vi "winchMotorCode.vi"() -> (2 "armMotorValue":dbl, 3 "elToroSplit":bool)   [LabVIEW 2013]
uses:
  <vilib>/Rock Robotics/WPI/DriverStation/WPI_DriverStationCommDataCacheOp.ctl
panel:
  in  "upperBoundDunk":dbl=16000.0
  in  "lowerBoundDunk":dbl=13000.0
  out "RawControlByte":u8 format="%08b"
  in  "upperBoundTruss":dbl=13000.0 format="%#_13g"
  in  "lowerBoundTruss":dbl=8000.0 format="%#_13g"
  in  "Encoder height shot constant":dbl=18500.0 format="%#_13g"
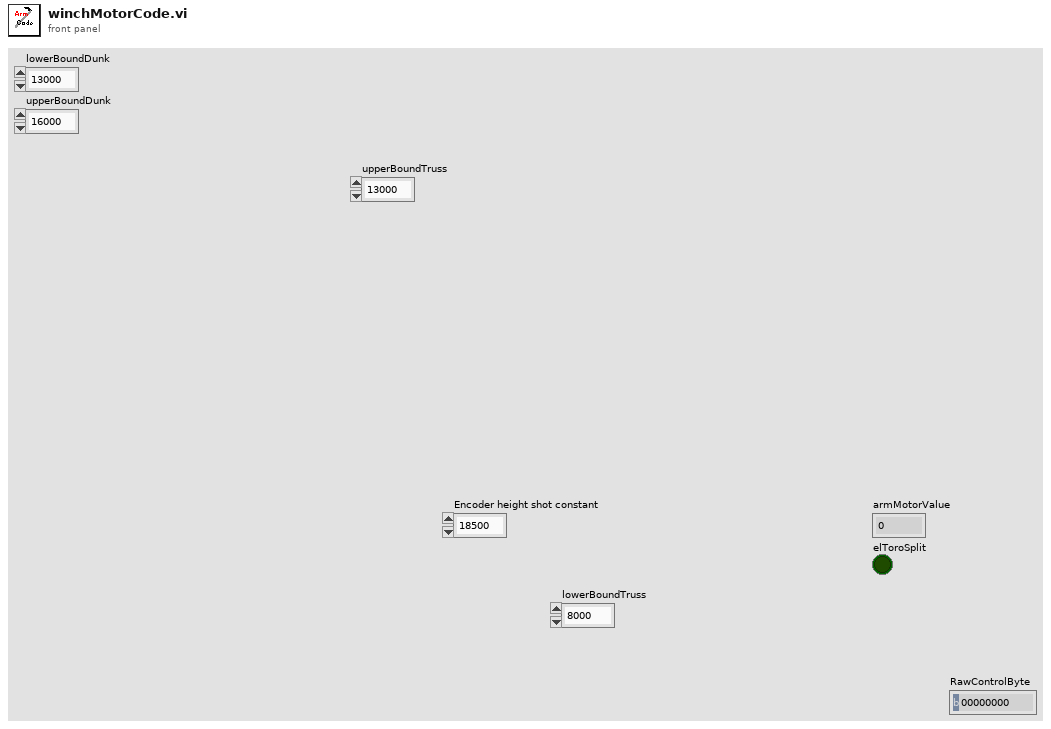
[diagram p1: front panel]
types:
  T1 = typedef "WPI_DriverStationCommDataCacheOp.ctl" = enum16{"Get", "Set", "Init"}
  T2 = typedef "WPI_EncoderDevRef.ctl" = cluster{"DevStatus":errorcluster, "EncoderIndex":T3, "CounterIndex":T4, "DistancePerCount":dbl, "Decoding Type":T5}
  T3 = typedef "FPGA_EncoderIdx.ctl" = enum8{"Enc 0", "Enc 1", "Enc 2", "Enc 3", "Invalid"}
  T4 = typedef "FPGA_CounterCtrSystemIndex.ctl" = enum8{"Ctr 0", "Ctr 1", "Ctr 2", "Ctr 3", "Ctr 4", "Ctr 5", "Ctr 6", "Ctr 7", "Invalid"}
  T5 = typedef "WPI_EncoderType.ctl" = enum16{"1x", "2x", "4x"}
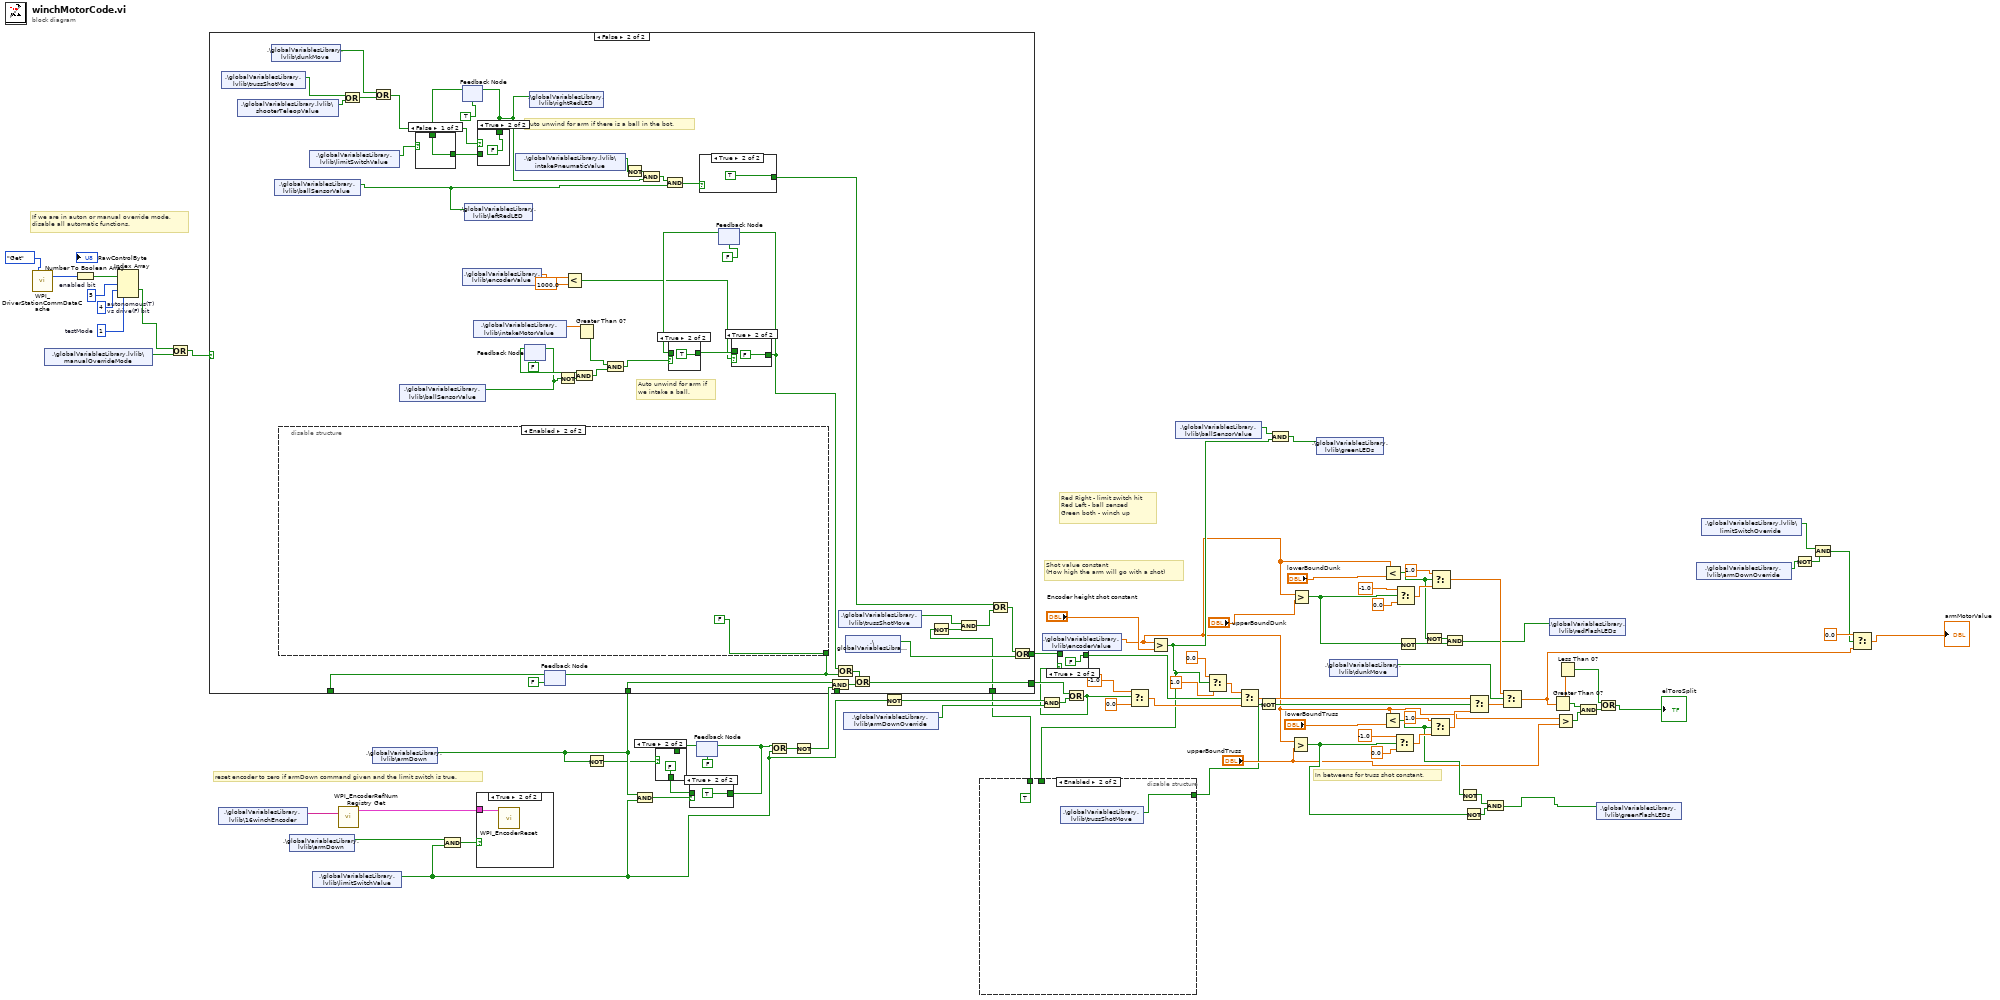
[diagram p0: block diagram]
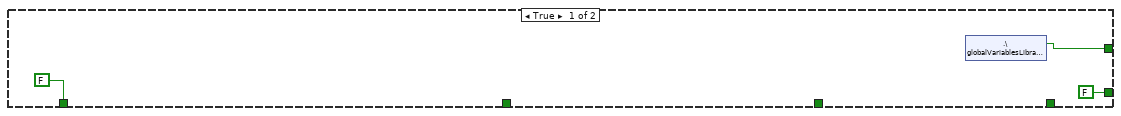
[diagram p2: hidden frame]
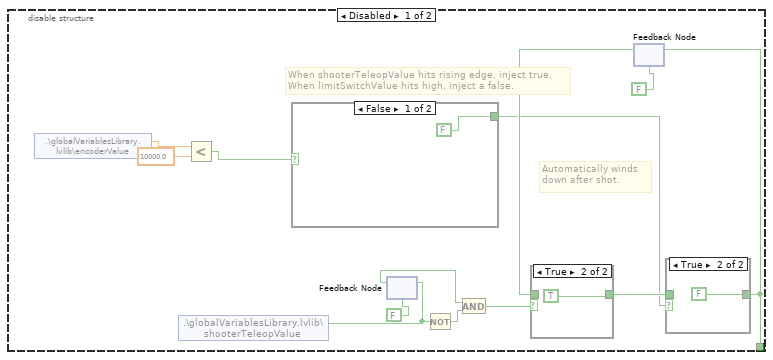
[diagram p3: hidden frame]
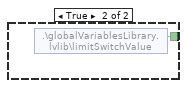
[diagram p4: hidden frame]
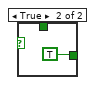
[diagram p10: hidden frame]
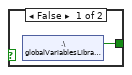
[diagram p11: hidden frame]
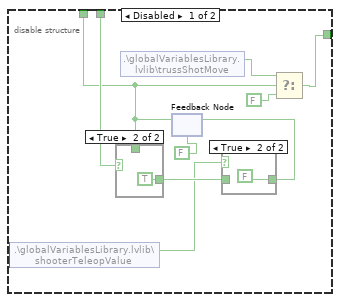
[diagram p12: hidden frame]
diagram:
  w29 = 1  # testMode
  w30 = 4  # autonomous(T) vs drive(F) bit
  w31 = 5  # enabled bit
  # "If we are in auton or manual override mode,\ndisable all automatic functions."
  # "reset encoder to zero if armDown command given and the limit switch is true."
  # "Red Right - limit switch hit\nRed Left - ball sensed\nGreen both - winch up"
  # "In betweens for truss shot constant."
  # "Shot value constant\n(How high the arm will go with a shot)"
  n1 = call <vilib>:"WPI_DriverStationCommDataCache.vi"("CommDataCacheOp"=WPI_DriverStationCommDataCacheOp."Get") -> ("ControlBit out"=w33:u8)  [unwired: 18 out]
  n2 = shared-variable ".\\globalVariablesLibrary.lvlib\\manualOverrideMode"() -> (w26:bool)  [unwired: 1 in, 1 out]
  n3 = Number To Boolean Array(number=w33) -> (Boolean array=w32:bool[])
  n4 = Index Array(array=w32, index #1=w31, index #2=w30, index #3=w29) -> (element #2=w24:bool)  [unwired: 2 out]
  n5 = Or(x=w24, y=w26) -> (x .or. y?=w25:bool)
  n6 = shared-variable ".\\globalVariablesLibrary.lvlib\\16winchEncoder"() -> (w74:string)  [unwired: 1 in, 1 out]
  n7 = shared-variable ".\\globalVariablesLibrary.lvlib\\armDown"() -> (w1:bool)  [unwired: 1 in, 1 out]
  n8 = shared-variable ".\\globalVariablesLibrary.lvlib\\limitSwitchValue"() -> (w38:bool)  [unwired: 1 in, 1 out]
  n9 = call <vilib>:"WPI_EncoderRefNum Registry Get.vi"("refnum name"=w74) -> ("EncoderDevRef"=w75:T2)  [unwired: 9 in, 1 out]
  n10 = shared-variable ".\\globalVariablesLibrary.lvlib\\armDown"() -> (w55:bool)  [unwired: 1 in, 1 out]
  n11 = And(x=w1, y=w38) -> (x .and. y?=w63:bool)
  n12 = case shown="True" w63 {
    tunnel: w75 -> [_ w84]
    frame False {
    }
    frame True {
      n13 = call <vilib>:"WPI_EncoderReset.vi"("EncoderDevRef"=w84) -> ()  [unwired: 9 in, 2 out]
    }
  }
  n14 = Not(x=w55) -> (.not. x?=w49:bool)
  n15 = And(x=w55, y=w38) -> (x .and. y?=w68:bool)
  n16 = feedback #1(FALSE) -> (w65:bool)
  n17 = case shown="True" w49 {
    tunnel: [w85 FALSE] -> w66
    tunnel: w65 -> [w85 _]
    frame False {
    }
    frame True {
    }
  }
  n18 = case shown="True" w68 {
    tunnel: [w87 TRUE] -> w64
    tunnel: w66 -> [w87 _]
    frame False {
    }
    frame True {
    }
  }
  n19 = feedback-in #1(w64) -> ()
  n20 = Or(x=w64, y=w38) -> (x .or. y?=w57:bool)
  n21 = Not(x=w57) -> (.not. x?=w56:bool)
  n22 = shared-variable ".\\globalVariablesLibrary.lvlib\\armDownOverride"() -> (w51:bool)  [unwired: 1 in, 1 out]
  n23 = Not(x=w38) -> (.not. x?=w52:bool)
  n24 = And(x=w52, y=w51) -> (x .and. y?=w53:bool)
  n25 = shared-variable ".\\globalVariablesLibrary.lvlib\\encoderValue"() -> (w13:dbl)  [unwired: 1 in, 1 out]
  n26 = Greater?(x=w13, y="Encoder height shot constant") -> (0:w36:bool)
  n27 = disable-structure shown="Enabled" {
    disable-tunnel: [w94 w102] -> w37
    disable-tunnel: w36 -> [w91 _]
    disable-tunnel: [w89 TRUE] -> w35
    frame Disabled {
      n28 = shared-variable ".\\globalVariablesLibrary.lvlib\\shooterTeleopValue"() -> (w90:bool)  [unwired: 1 in, 1 out]
      n29 = shared-variable ".\\globalVariablesLibrary.lvlib\\trussShotMove"() -> (w92:bool)  [unwired: 1 in, 1 out]
      n30 = feedback #2(FALSE) -> (w89:bool)
      n31 = case shown="True" w91 {
        tunnel: [w100 TRUE] -> w97
        tunnel: w89 -> [w100 _]
        frame False {
        }
        frame True {
        }
      }
      n32 = case shown="True" w90 {
        tunnel: [w98 FALSE] -> w96
        tunnel: w97 -> [w98 _]
        frame False {
        }
        frame True {
        }
      }
      n33 = feedback-in #2(w96) -> ()
      n34 = Select(t=w92, s=w89, f=FALSE) -> (s? t:f=w94:bool)
    }
    frame Enabled {
      n35 = shared-variable ".\\globalVariablesLibrary.lvlib\\trussShotMove"() -> (w102:bool)  [unwired: 1 in, 1 out]
    }
  }
  n36 = case shown="False" w25 {
    tunnel: w56 -> [_ w146]
    tunnel: w55 -> [_ w145]
    tunnel: [FALSE w144] -> w54
    tunnel: [FALSE w135] -> _
    tunnel: [w106 w116] -> w46
    tunnel: w35 -> [_ w110]
    frame True {
      n37 = shared-variable ".\\globalVariablesLibrary.lvlib\\armUp"() -> (w106:bool)  [unwired: 1 in, 1 out]
    }
    frame False {
      # "Auto unwind for arm if we intake a ball."
      # "Auto unwind for arm if there is a ball in the bot."
      n38 = shared-variable ".\\globalVariablesLibrary.lvlib\\trussShotMove"() -> (w136:bool)  [unwired: 1 in, 1 out]
      n39 = shared-variable ".\\globalVariablesLibrary.lvlib\\shooterTeleopValue"() -> (w137:bool)  [unwired: 1 in, 1 out]
      n40 = shared-variable ".\\globalVariablesLibrary.lvlib\\dunkMove"() -> (w107:bool)  [unwired: 1 in, 1 out]
      n41 = shared-variable ".\\globalVariablesLibrary.lvlib\\ballSensorValue"() -> (w138:bool)  [unwired: 1 in, 1 out]
      n42 = disable-structure shown="Enabled" {
        disable-tunnel: [w153 FALSE] -> w120
        frame Disabled {
          # "Automatically winds down after shot."
          # "When shooterTeleopValue hits rising edge, inject true.\nWhen limitSwitchValue hits high, inject a false."
          n43 = shared-variable ".\\globalVariablesLibrary.lvlib\\encoderValue"() -> (w156:dbl)  [unwired: 1 in, 1 out]
          n44 = shared-variable ".\\globalVariablesLibrary.lvlib\\shooterTeleopValue"() -> (w160:bool)  [unwired: 1 in, 1 out]
          n45 = Less?(x=w156, y=10000.0) -> (x < y?=w154:bool)
          n46 = case shown="False" w154 {
            tunnel: [FALSE w167] -> w158
            frame False {
            }
            frame True {
              n47 = shared-variable ".\\globalVariablesLibrary.lvlib\\limitSwitchValue"() -> (w167:bool)  [unwired: 1 in, 1 out]
            }
          }
          n48 = feedback #3(FALSE) -> (w159:bool)
          n49 = feedback-in #3(w160) -> ()
          n50 = Not(x=w160) -> (.not. x?=w161:bool)
          n51 = And(x=w159, y=w161) -> (x .and. y?=w157:bool)
          n52 = feedback #4(FALSE) -> (w164:bool)
          n53 = case shown="True" w157 {
            tunnel: [w170 TRUE] -> w163
            tunnel: w164 -> [w170 _]
            frame False {
            }
            frame True {
            }
          }
          n54 = case shown="True" w158 {
            tunnel: w163 -> [w168 _]
            tunnel: [w168 FALSE] -> w153
            frame False {
            }
            frame True {
            }
          }
          n55 = feedback-in #4(w153) -> ()
        }
        frame Enabled {
        }
      }
      n56 = shared-variable ".\\globalVariablesLibrary.lvlib\\limitSwitchValue"() -> (w150:bool)  [unwired: 1 in, 1 out]
      n57 = Or(x=w136, y=w137) -> (x .or. y?=w109:bool)
      n58 = Or(x=w107, y=w109) -> (x .or. y?=w108:bool)
      n59 = shared-variable ".\\globalVariablesLibrary.lvlib\\ballSensorValue"() -> (w132:bool)  [unwired: 1 in, 1 out]
      n60 = feedback #5(TRUE) -> (w149:bool)
      n61 = case shown="False" w150 {
        tunnel: w149 -> [w179 _]
        tunnel: [w179 TRUE] -> w148
        frame False {
        }
        frame True {
        }
      }
      n62 = shared-variable ".\\globalVariablesLibrary.lvlib\\encoderValue"() -> (w123:dbl)  [unwired: 1 in, 1 out]
      n63 = shared-variable ".\\globalVariablesLibrary.lvlib\\leftRedLED"(w138) -> ()  [unwired: 1 in, 1 out]
      n64 = shared-variable ".\\globalVariablesLibrary.lvlib\\intakeMotorValue"() -> (w118:dbl)  [unwired: 1 in, 1 out]
      n65 = case shown="True" w108 {
        tunnel: w148 -> [w177 _]
        tunnel: [w177 FALSE] -> w142
        frame False {
        }
        frame True {
        }
      }
      n66 = feedback-in #5(w142) -> ()
      n67 = shared-variable ".\\globalVariablesLibrary.lvlib\\intakePneumaticValue"() -> (w140:bool)  [unwired: 1 in, 1 out]
      n68 = feedback #6(FALSE ("Boolean")) -> (w133:bool)
      n69 = feedback-in #6(w132) -> ()
      n70 = shared-variable ".\\globalVariablesLibrary.lvlib\\rightRedLED"(w142) -> ()  [unwired: 1 in, 1 out]
      n71 = feedback #7(FALSE) -> (w135:bool)
      n72 = feedback-in #7(w120) -> ()
      n73 = Not(x=w132) -> (.not. x?=w131:bool)
      n74 = Less?(x=w123, y=1000.0) -> (x < y?=w122:bool)
      n75 = And(x=w133, y=w131) -> (x .and. y?=w130:bool)
      n76 = Greater Than 0?(x=w118) -> (x > 0?=w117:bool)
      n77 = And(x=w117, y=w130) -> (x .and. y?=w126:bool)
      n78 = Not(x=w140) -> (.not. x?=w141:bool)
      n79 = And(x=w141, y=w142) -> (x .and. y?=w143:bool)
      n80 = And(x=w143, y=w138) -> (x .and. y?=w151:bool)
      n81 = case shown="True" w151 {
        tunnel: [w181 TRUE] -> w115
        frame False {
          n82 = shared-variable ".\\globalVariablesLibrary.lvlib\\armUp"() -> (w181:bool)  [unwired: 1 in, 1 out]
        }
        frame True {
        }
      }
      n83 = feedback #8(FALSE) -> (w125:bool)
      n84 = case shown="True" w126 {
        tunnel: [w175 TRUE] -> w127
        tunnel: w125 -> [w175 _]
        frame False {
        }
        frame True {
        }
      }
      n85 = case shown="True" w122 {
        tunnel: w127 -> [w173 _]
        tunnel: [w173 FALSE] -> w119
        frame False {
        }
        frame True {
        }
      }
      n86 = feedback-in #8(w119) -> ()
      n87 = And(x=w145, y=w146) -> (x .and. y?=w147:bool)
      n88 = Or(x=w119, y=w120) -> (x .or. y?=w121:bool)
      n89 = shared-variable ".\\globalVariablesLibrary.lvlib\\trussShotMove"() -> (w111:bool)  [unwired: 1 in, 1 out]
      n90 = shared-variable ".\\globalVariablesLibrary.lvlib\\armUp"() -> (w139:bool)  [unwired: 1 in, 1 out]
      n91 = Or(x=w121, y=w147) -> (x .or. y?=w144:bool)
      n92 = Not(x=w110) -> (.not. x?=w112:bool)
      n93 = And(x=w111, y=w112) -> (x .and. y?=w113:bool)
      n94 = Or(x=w115, y=w113) -> (x .or. y?=w114:bool)
      n95 = Or(x=w114, y=w139) -> (x .or. y?=w116:bool)
    }
  }
  n96 = Or(x=w54, y=w53) -> (x .or. y?=w2:bool)
  n97 = case shown="True" w2 {
    tunnel: w46 -> [w183 _]
    tunnel: [w183 FALSE] -> w45
    frame False {
    }
    frame True {
    }
  }
  n98 = Select(t=-1.0, s=w2, f=0.0) -> (s? t:f=w58:dbl)
  n99 = shared-variable ".\\globalVariablesLibrary.lvlib\\ballSensorValue"() -> (w48:bool)  [unwired: 1 in, 1 out]
  n100 = Select(t=0.0, s=w36, f=1.0) -> (s? t:f=w71:dbl)
  n101 = Select(t=w71, s=w45, f=w58) -> (s? t:f=w76:dbl)
  n102 = Not(x=w37) -> (.not. x?=w77:bool)
  n103 = And(x=w48, y=w36) -> (x .and. y?=w47:bool)
  n104 = Greater?(x=w13, y="upperBoundTruss") -> (0:w60:bool)
  n105 = Greater?(x=w13, y="upperBoundDunk") -> (0:w11:bool)
  n106 = shared-variable ".\\globalVariablesLibrary.lvlib\\greenLEDs"(w47) -> ()  [unwired: 1 in, 1 out]
  n107 = shared-variable ".\\globalVariablesLibrary.lvlib\\dunkMove"() -> (w7:bool)  [unwired: 1 in, 1 out]
  n108 = Less?(x=w13, y="lowerBoundTruss") -> (x < y?=w61:bool)
  n109 = Less?(x=w13, y="lowerBoundDunk") -> (x < y?=w12:bool)
  n110 = Select(t=-1.0, s=w60, f=0.0) -> (s? t:f=w80:dbl)
  n111 = Select(t=-1.0, s=w11, f=0.0) -> (s? t:f=w18:dbl)
  n112 = Not(x=w11) -> (.not. x?=w3:bool)
  n113 = Not(x=w12) -> (.not. x?=w4:bool)
  n114 = Select(t=1.0, s=w61, f=w80) -> (s? t:f=w83:dbl)
  n115 = Select(t=1.0, s=w12, f=w18) -> (s? t:f=w8:dbl)
  n116 = And(x=w4, y=w3) -> (x .and. y?=w5:bool)
  n117 = Not(x=w61) -> (.not. x?=w59:bool)
  n118 = Not(x=w60) -> (.not. x?=w62:bool)
  n119 = Select(t=w76, s=w77, f=w83) -> (s? t:f=w10:dbl)
  n120 = And(x=w59, y=w62) -> (x .and. y?=w6:bool)
  n121 = Select(t=w8, s=w7, f=w10) -> (s? t:f=w9:dbl)
  n122 = shared-variable ".\\globalVariablesLibrary.lvlib\\redFlashLEDs"(w5) -> ()  [unwired: 1 in, 1 out]
  n123 = Greater Than 0?(x=w9) -> (x > 0?=w44:bool)
  n124 = Greater?(x=w13, y="upperBoundTruss") -> (0:w43:bool)
  n125 = Less Than 0?(x=w9) -> (x < 0?=w39:bool)
  n126 = And(x=w44, y=w43) -> (x .and. y?=w41:bool)
  n127 = shared-variable ".\\globalVariablesLibrary.lvlib\\greenFlashLEDs"(w6) -> ()  [unwired: 1 in, 1 out]
  n128 = Or(x=w39, y=w41) -> (x .or. y?=→"elToroSplit":bool)
  n129 = shared-variable ".\\globalVariablesLibrary.lvlib\\armDownOverride"() -> (w21:bool)  [unwired: 1 in, 1 out]
  n130 = shared-variable ".\\globalVariablesLibrary.lvlib\\limitSwitchOverride"() -> (w23:bool)  [unwired: 1 in, 1 out]
  n131 = Not(x=w21) -> (.not. x?=w22:bool)
  n132 = And(x=w23, y=w22) -> (x .and. y?=w20:bool)
  n133 = Select(t=0.0 ("f"), s=w20, f=w9) -> (s? t:f=→"armMotorValue":dbl)
